vi "ADAM_Module_Type.vi"(1 "Module Type":T1) -> (0 "String":string)   [LabVIEW 2010]
uses:
  ADAM Controls/Module_type_ADAM.ctl
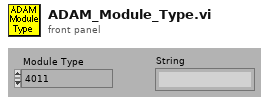
[diagram p1: front panel]
types:
  T1 = typedef "Module_type_ADAM.ctl" = enum16{"4011", "4012", "4013", "4014", "4016", "4017", "4018", "4021", "4050", "4052", "4053", "4060", "4080", "5000", "5017", "5018", "5024", "5051", "5056", "5060", "6060", "Tracker", "WEST", "GILL", "JEM", "VICI", "Vaisala", "DRUCK", "Run VI Named:", "IR2100", "PPT", "Comparator", "VIRTUAL", "Hold Value", "Read A", "Read Ch", "Coded", "Client Info", "Web Client", "X10", "Test"}
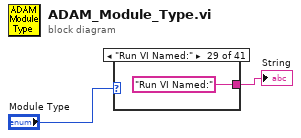
[diagram p0: block diagram]
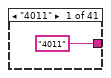
[diagram p2: hidden frame]
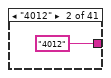
[diagram p3: hidden frame]
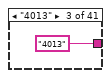
[diagram p4: hidden frame]
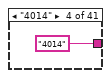
[diagram p5: hidden frame]
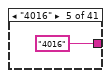
[diagram p6: hidden frame]
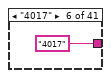
[diagram p7: hidden frame]
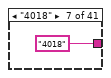
[diagram p8: hidden frame]
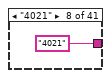
[diagram p9: hidden frame]
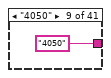
[diagram p10: hidden frame]
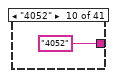
[diagram p11: hidden frame]
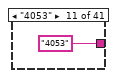
[diagram p12: hidden frame]
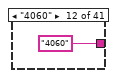
[diagram p13: hidden frame]
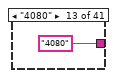
[diagram p14: hidden frame]
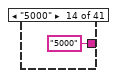
[diagram p15: hidden frame]
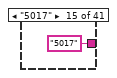
[diagram p16: hidden frame]
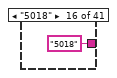
[diagram p17: hidden frame]
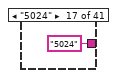
[diagram p18: hidden frame]
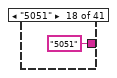
[diagram p19: hidden frame]
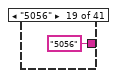
[diagram p20: hidden frame]
diagram:
  n1 = case shown="\"Run VI Named:\"" "Module Type" {
    tunnel: ["4011" "4012" "4013" "4014" "4016" "4017" "4018" "4021" "4050" "4052" "4053" "4060" "4080" "5000" "5017" "5018" "5024" "5051" "5056" "5060" "6060" "Tracker" "WEST" "GILL" "JEM" "VICI" "Vaisala" "DRUCK" "Run VI Named:" "IR2100" "PPT" "Comparator" "VIRTUAL" "Coded" "Client Info" "Web Client" "Read A" "Read Ch" "Hold Value" "X10" "Test"] -> w2
    frame "4011" {
    }
    frame "4012" {
    }
    frame "4013" {
    }
    frame "4014" {
    }
    frame "4016" {
    }
    frame "4017" {
    }
    frame "4018" {
    }
    frame "4021" {
    }
    frame "4050" {
    }
    frame "4052" {
    }
    frame "4053" {
    }
    frame "4060" {
    }
    frame "4080" {
    }
    frame "5000" {
    }
    frame "5017" {
    }
    frame "5018" {
    }
    frame "5024" {
    }
    frame "5051" {
    }
    frame "5056" {
    }
    frame "5060" {
    }
    frame "6060" {
    }
    frame "Tracker" {
    }
    frame "WEST" {
    }
    frame "GILL" {
    }
    frame "JEM" {
    }
    frame "VICI" {
    }
    frame "Vaisala" {
    }
    frame "DRUCK" {
    }
    frame "Run VI Named:" {
    }
    frame "IR2100" {
    }
    frame "PPT" {
    }
    frame "Comparator" {
    }
    frame "VIRTUAL" {
    }
    frame "Coded" {
    }
    frame "Client Info" {
    }
    frame "Web Client" {
    }
    frame "Read A" {
    }
    frame "Read Ch" {
    }
    frame "Hold Value" {
    }
    frame "X10" {
    }
    frame "Test" {
    }
  }
  "String" <- w2
